vi "Push Synchronized Analog.vi"(9 "samples chn 2":dbl[](array[numeric]), 10 "samples chn 1":dbl[](array[numeric]), 11 "ADALM2000 Handler":u32 caption="Instrument Handle Out") -> (3 "ADALM2000 Handler 2":u32 caption="Instrument Handle Out")   [LabVIEW 2015]
uses:
  libm2k_lv.dll
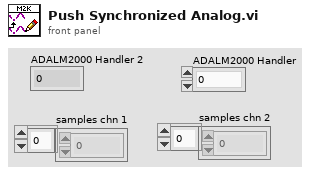
[diagram p1: front panel]
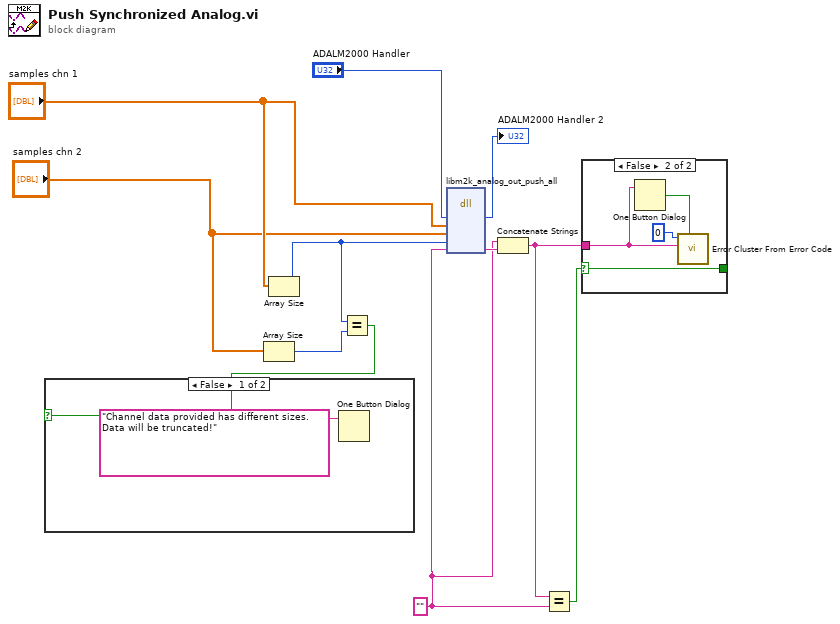
[diagram p0: block diagram]
diagram:
  w7 = ""
  n1 = Array Size(array="samples chn 2") -> (size(s)=w2:i32)
  n2 = Array Size(array="samples chn 1") -> (size(s)=w3:i32)
  n3 = Equal?(x=w3, y=w2) -> (x = y?=w1:bool)
  n4 = case shown="False" w1 {
    frame False {
      n5 = One Button Dialog(message="Channel data provided has different sizes. Data will be truncated!") -> ()  [unwired: 1 in, 1 out]
    }
    frame True {
    }
  }
  n6 = dll-call lib="libm2k_lv.*" fn="libm2k_analog_out_push_all"("instance"="ADALM2000 Handler", "samples_ch1"="samples chn 1", "samples_ch2"="samples chn 2", "nb_samples_per_chn"=w3, "err"=w7) -> ("instance"=→"ADALM2000 Handler 2":u64, "err"=w10:string)  [unwired: 7 in, 2 out]
  n7 = Concatenate Strings(w7, w10) -> (w6:string)
  n8 = Equal?(x=w6, y=w7) -> (x = y?=w5:bool)
  n9 = case shown="False" w5 {
    selector: w5 -> [w13 w14]
    tunnel: w6 -> [_ w16]
    tunnel: [w13 w14] -> _
    frame True {
    }
    frame False {
      n10 = One Button Dialog(message=w16) -> (true=w15:bool)  [unwired: 1 in]
      n11 = call <vilib>:"Error Cluster From Error Code.vi"("show call chain? (False)"=w15, "error message (\"\")"=w16, "error code (0)"=0) -> ()  [unwired: 6 in, 1 out]
    }
  }
